vi "top_level.vi"(10 "progress ref":refnum<vi>, 11 "series URL":string) -> (0 "error out":errorcluster, 3 "seriesInfo":T2)   [LabVIEW 2024]
uses:
  series_class/seriesInfo--cluster.ctl
  comic_class/issueInfo--cluster.ctl
  comic_class/creator--cluster.ctl
  comic_class/character--cluster.ctl
  comic_class/team--cluster.ctl
  comic_class/location--cluster.ctl
  comic_class/concept--cluster.ctl
  comic_class/thing--cluster.ctl
  comic_class/storyArc--cluster.ctl
  series_class/seriesJSON--cluster.ctl
  series_class/series_class.lvclass
  C:/code/LabVIEW_Projects/applications/ComicVine_API/WebScraper/comic_class/comic_class.lvclass
  series_class/series_class.lvclass/series_class.ctl
  <vilib>/Utility/High Resolution Relative Seconds.vi
  comic_class/comic_class.lvclass
  <vilib>/addons/_JKI.lib/Serialization/JSON/JKI JSON Serialization.lvlib
  C:/code/LabVIEW_Projects/applications/ComicVine_API/WebScraper/series_class/series_class.lvclass
panel:
  in  "output cluster":T1
  out "issues":T3[](array[typedef])
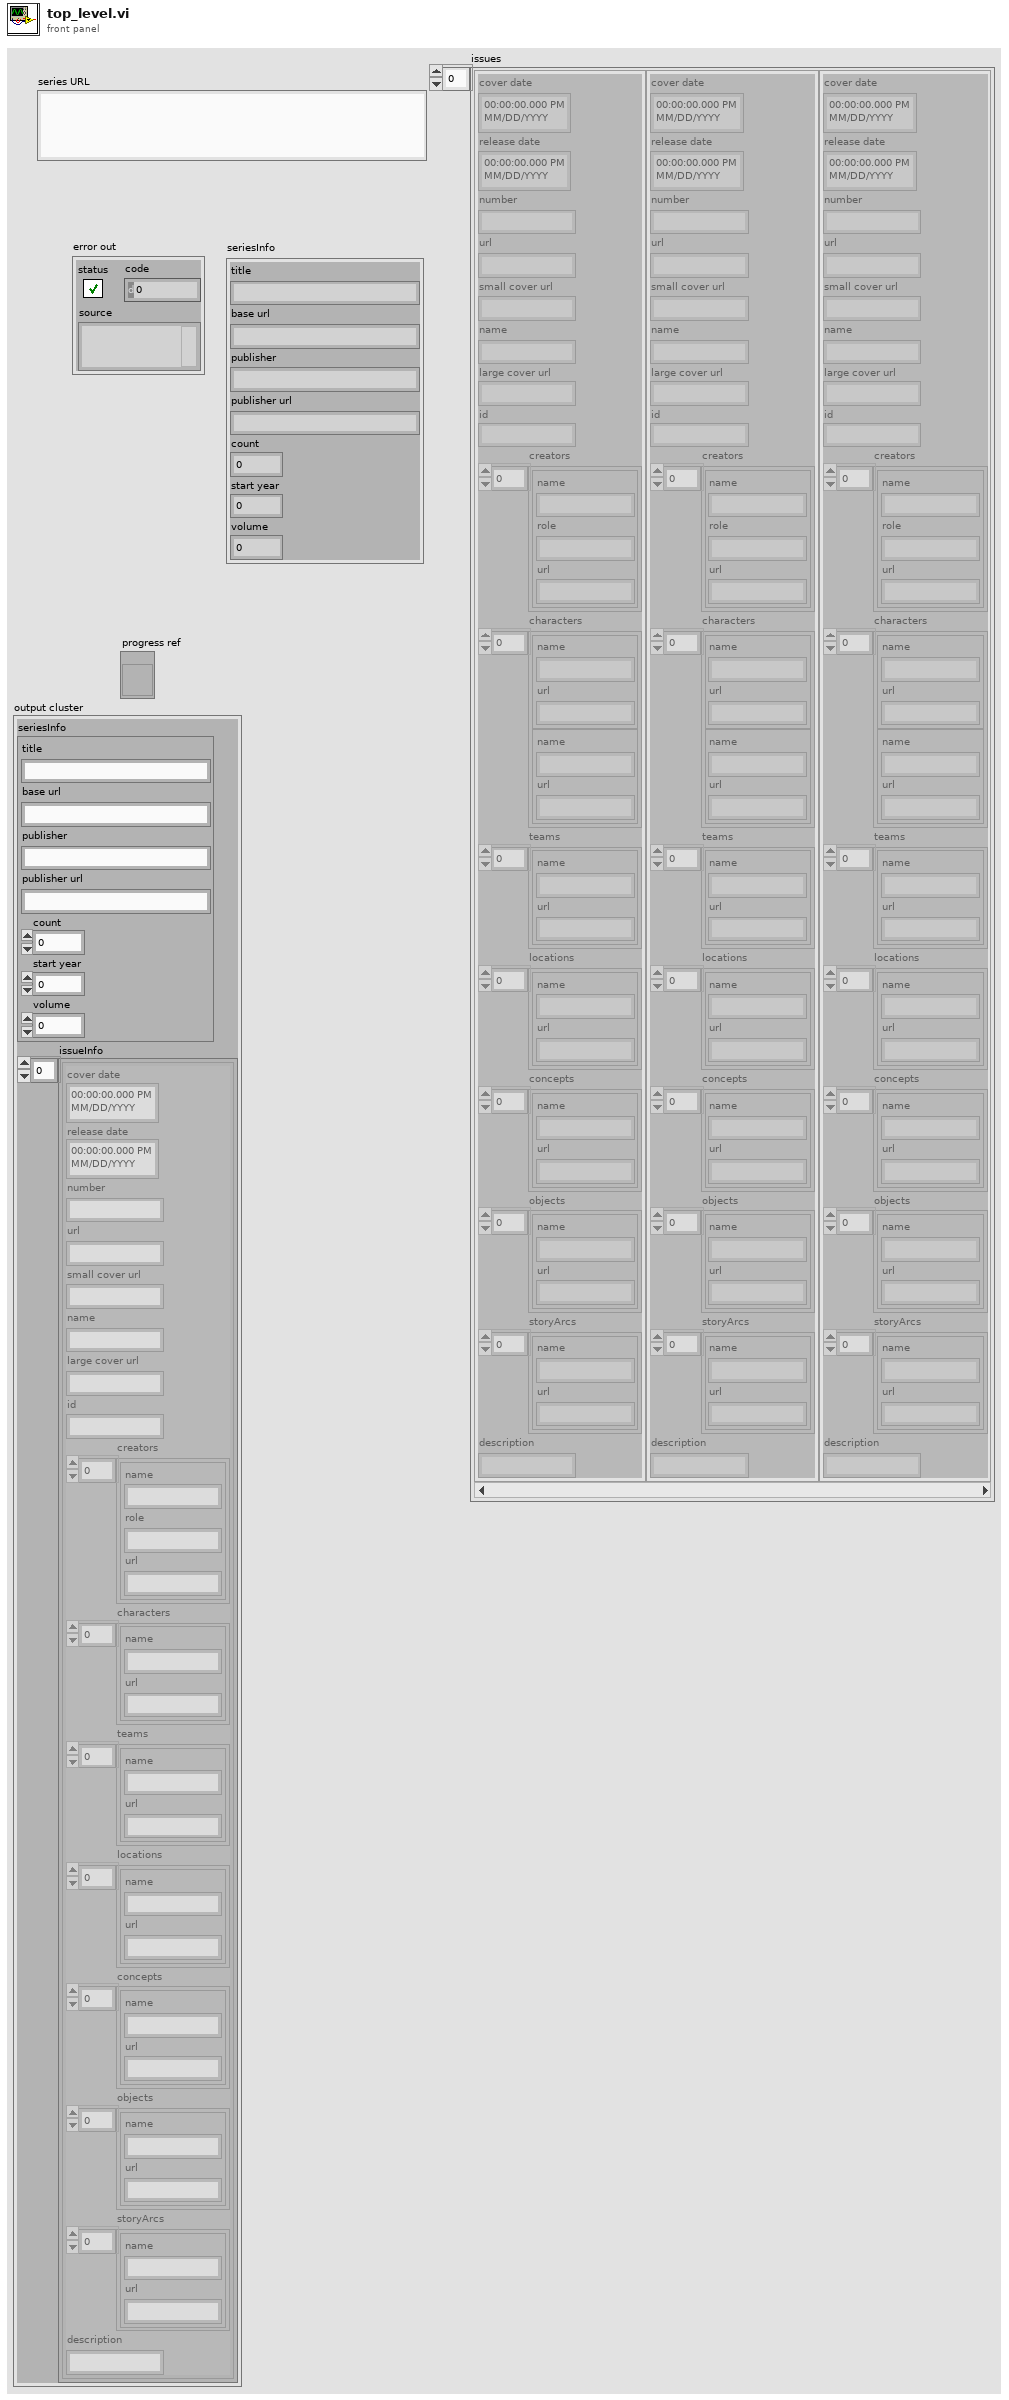
[diagram p1: front panel]
types:
  T1 = typedef "series_class.lvclass/seriesJSON--cluster.ctl" = cluster{"seriesInfo":T2, "issueInfo":T3[]}
  T2 = typedef "series_class.lvclass/seriesInfo--cluster.ctl" = cluster{"title":string, "base url":string, "publisher":string, "publisher url":string, "count":i32, "start year":i32, "volume":i32}
  T3 = typedef "comic_class.lvclass/issueInfo--cluster.ctl" = cluster{"cover date":timestamp, "release date":timestamp, "number":string, "url":string, "small cover url":string, "name":string, "large cover url":string, "id":string, "creators":T4[], "characters":T5[], "teams":T6[], "locations":T7[], "concepts":T8[], "objects":T9[], "storyArcs":T10[], "description":string}
  T4 = typedef "comic_class.lvclass/creator--cluster.ctl" = cluster{"name":string, "role":string, "url":string}
  T5 = typedef "comic_class.lvclass/character--cluster.ctl" = cluster{"name":string, "url":string}
  T6 = typedef "comic_class.lvclass/team--cluster.ctl" = cluster{"name":string, "url":string}
  T7 = typedef "comic_class.lvclass/location--cluster.ctl" = cluster{"name":string, "url":string}
  T8 = typedef "comic_class.lvclass/concept--cluster.ctl" = cluster{"name":string, "url":string}
  T9 = typedef "comic_class.lvclass/thing--cluster.ctl" = cluster{"name":string, "url":string}
  T10 = typedef "comic_class.lvclass/storyArc--cluster.ctl" = cluster{"name":string, "url":string}
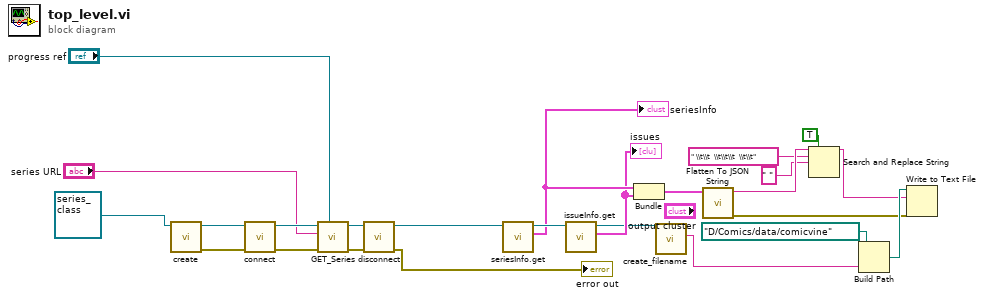
[diagram p0: block diagram]
diagram:
  n1 = call "create.vi"("comic_class in"=refnum<class "series_class.lvclass"> refnum ("series_class.lvclass")) -> ("error out"=w25:errorcluster, "comic_class out"=w24:refnum<class "series_class.lvclass">)  [unwired: 9 in]
  n2 = call-dynamic "connect.vi"("error in (no error)"=w25, "comic_class in"=w24) -> ("error out"=w20:errorcluster, "comic_class out"=w21:refnum<class "series_class.lvclass">)  [unwired: 8 in]
  n3 = call "GET_Series.vi"("progress ref"="progress ref", "error in (no error)"=w20, "series URL"="series URL", "ComicVine_class in"=w21) -> ("error out"=w22:errorcluster, "ComicVine_class out"=w23:refnum<class "series_class.lvclass">)  [unwired: 6 in]
  n4 = call-dynamic "disconnect.vi"("error in (no error)"=w22, "comic_class in"=w23) -> ("error out"=→"error out":errorcluster, "comic_class out"=w19:refnum<class "series_class.lvclass">)  [unwired: 8 in]
  n5 = call "seriesInfo.get.vi"("ComicVine_class in"=w19) -> ("seriesInfo"=w16:T2, "ComicVine_class out"=w18:refnum<class "series_class.lvclass">)  [unwired: 9 in]
  "seriesInfo" <- w16
  n6 = call "issueInfo.get.vi"("ComicVine_class in"=w18) -> ("issueInfo"=w15:T3[], "ComicVine_class out"=w10:refnum<class "series_class.lvclass">)  [unwired: 9 in]
  "issues" <- w15
  n7 = Bundle("seriesInfo"=w16, "issueInfo"=w15) -> (w14:cluster{"seriesInfo":T2, "issueInfo":T3[]})  [unwired: 1 in]
  n8 = call "create_filename.vi"("series_class in"=w10) -> ("json filename"=w9:string)  [unwired: 9 in, 1 out]
  n9 = call <vilib>:"Flatten To JSON String.vi"("Variant"=w14) -> ("error out"=w11:errorcluster, "JSON String"=w8:string)  [unwired: 9 in]
  n10 = Search and Replace String(replace all?=TRUE ("replace all? (F)"), input string=w8, search string=" \\t\\t  \\t\\t\\t  \\t\\t", replace string=" " ("replace string (\"\")")) -> (result string=w7:string)  [unwired: 4 in, 3 out]
  n11 = Build Path(base path=path "D:/Comics/data/comicvine", name or relative path=w9) -> (appended path=w12:path)
  n12 = Write to Text File(file (use dialog)=w12, text=w7, error in=w11) -> ()  [unwired: 1 in, 3 out]
